vi "encryption.vi"(11 "字符串":string) -> (3 "转换值":string)   [LabVIEW 2019, in "User Management Model.lvclass"]
uses:
  User Management Model.lvclass
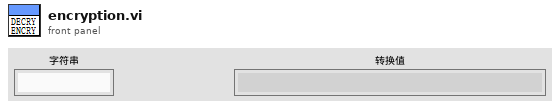
[diagram p1: front panel]
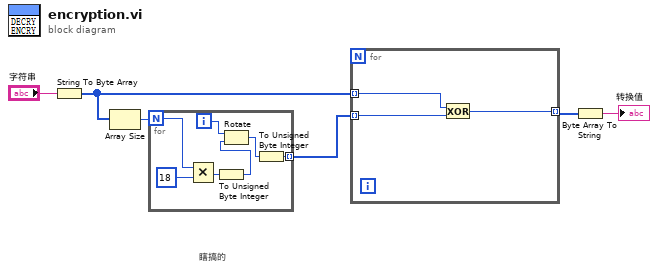
[diagram p0: block diagram]
diagram:
  # "瞎搞的"
  n1 = String To Byte Array(string="字符串") -> (unsigned byte array=w6:u8[])
  n2 = Array Size(array=w6) -> (size(s)=w5:i32)
  n3 = for {
    N: w5 -> [w11]
    tunnel: [w13] -> w2 mode=indexing
    i -> [w10]
    n4 = Multiply(x=w11, y=u8 18) -> (x*y=w8:i32)
    n5 = To Unsigned Byte Integer(number=w8) -> (unsigned 8bit integer=w7:u8)
    n6 = Rotate(1:w7, 2:w10) -> (0:w9:u8)
    n7 = To Unsigned Byte Integer(number=w9) -> (unsigned 8bit integer=w13:u8)
  }
  n8 = for {
    tunnel: w6 -> [w16] mode=indexing
    tunnel: w2 -> [w15] mode=indexing
    tunnel: [w14] -> w4 mode=indexing
    n9 = Exclusive Or(1:w15, 2:w16) -> (0:w14:u8)
  }
  n10 = Byte Array To String(unsigned byte array=w4) -> (string=→"转换值":string)
